vi "Initialise Kohrah.vi"(8 "error in (no error)":errorcluster, 11 "Renderer":u32) -> (0 "error out":errorcluster, 3 "Ship out":refnum<class "Kohrah.lvclass">)   [LabVIEW 2021, in "Kohrah.lvclass"]
uses:
  Kohrah.lvclass
  Ship/Config.ctl
  Ship/Ship.lvclass
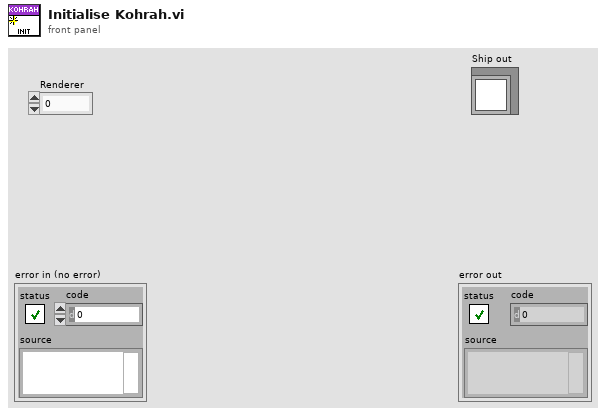
[diagram p1: front panel]
types:
  T1 = typedef "Ship.lvclass/Config.ctl" = cluster{"Race":string, "Ship Name":string, "Max Crew":i32, "Max Energy":i32, "Energy Regeneration":i32, "Weapon Energy Cost":i32, "Special Energy Cost":i32, "Energy Wait":i32, "Max Thrust":i32, "Thrust Increment":i32, "Turn Wait":i32, "Thrust Wait":i32, "Weapon Wait":i32, "Special Wait":i32, "Ship Mass":i32}
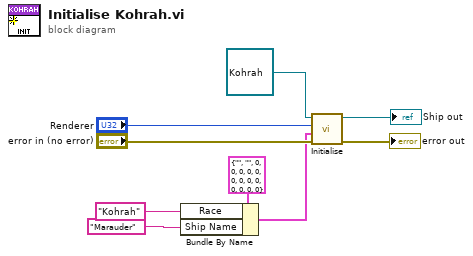
[diagram p0: block diagram]
diagram:
  n1 = Bundle By Name(cluster=T1 {"Race"="", "Ship Name"="", "Max Crew"=0, "Max Energy"=0, "Energy Regeneration"=0, "Weapon Energy Cost"=0, "Special Energy Cost"=0, "Energy Wait"=0, "Max Thrust"=0, "Thrust Increment"=0, "Turn Wait"=0, "Thrust Wait"=0, "Weapon Wait"=0, "Special Wait"=0, "Ship Mass"=0} ("Common"), "Race"="Kohrah" ("name or relative path"), "Ship Name"="Marauder") -> (w7:T1)
  n2 = call-dynamic "Initialise.vi"("error in (no error)"="error in (no error)", "Common"=w7, "Renderer"="Renderer", "Ship in"=refnum<class "Kohrah.lvclass"> refnum ("Ship")) -> ("error out"=→"error out":errorcluster, "Ship out"=→"Ship out":refnum<class "Kohrah.lvclass">)  [unwired: 6 in]
